vi "String to TimeStamp2012.vi"(0 "String in HH:MM:SS format":string="17:47:00") -> (6 "Time difference (sec)":dbl, 10 "String converted to Time Stamp":timestamp, 15 "Current Time":timestamp)   [LabVIEW 2012]
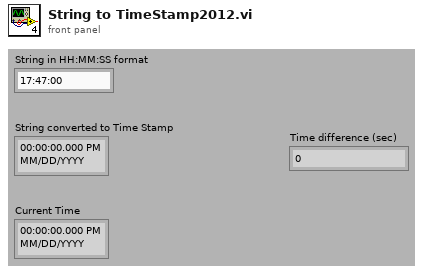
[diagram p1: front panel]
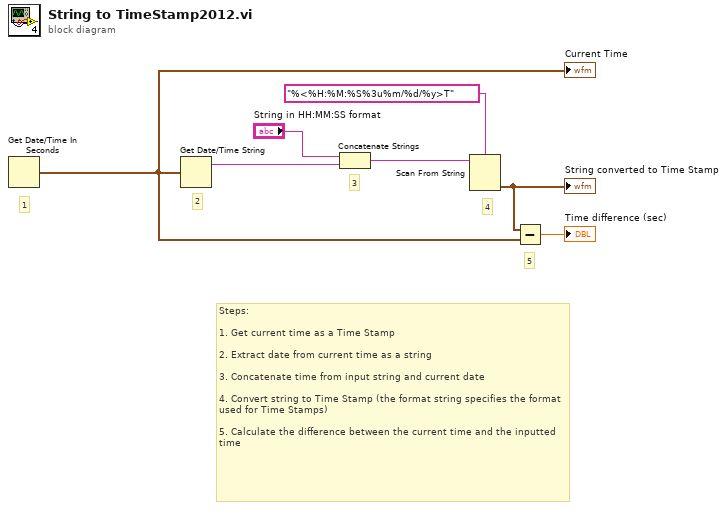
[diagram p0: block diagram]
diagram:
  # "5"
  # "4"
  # "3"
  # "2"
  # "1"
  # "Steps:\n\n1. Get current time as a Time Stamp\n\n2. Extract date from current time as a string\n\n3. Concatenate time from input string and current date\n \n4. Convert string to Time Stamp (the format string specifies the format used for Time Stamps)\n\n5. Calculate the difference between the current time and the inputted time"
  n1 = Get Date/Time In Seconds() -> (seconds since 1Jan1904=w3:timestamp)
  "Current Time" <- w3
  n2 = Get Date/Time String(seconds (now)=w3) -> (date string=w1:string)  [unwired: 3 out]
  n3 = Concatenate Strings "Concatenate Strings"("String in HH:MM:SS format", w1) -> (w5:string)
  n4 = Scan From String "Scan From String"(format string="%<%H:%M:%S%3u%m/%d/%y>T" ("input string"), input string=w5) -> (output 1=w4:timestamp)  [unwired: 2 in, 4 out]
  "String converted to Time Stamp" <- w4
  n5 = Subtract(x=w4, y=w3) -> (x-y=→"Time difference (sec)":dbl)
